vi "Manipulator Set Step.vi"(8 "error in (no error)":errorcluster, 10 "Step":i32, 11 "VISA resource in":refnum<visa-resource-name>="COM1") -> (0 "error out":errorcluster, 2 "Response":string, 3 "VISA resource out":refnum<visa-resource-name>)   [LabVIEW 2012, in "Scientifica Manipulator Daemon.lvlib"]
uses:
  Scientifica Manipulator Daemon.lvlib
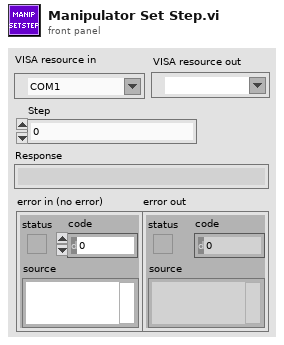
[diagram p1: front panel]
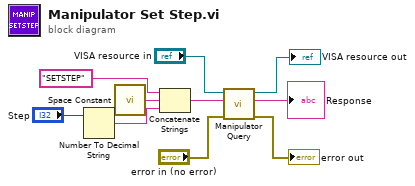
[diagram p0: block diagram]
diagram:
  n1 = Number To Decimal String(number="Step") -> (decimal integer string=w4:string)  [unwired: 1 in]
  n2 = call <vilib>:"Space Constant.vi"() -> ("String"=w5:string)
  n3 = Concatenate Strings("SETSTEP", w5, w4) -> (w3:string)
  n4 = call "Manipulator Query.vi"("error in (no error)"="error in (no error)", "Command"=w3, "VISA resource in"="VISA resource in") -> ("error out"=→"error out":errorcluster, "Response"=→"Response":string, "VISA resource out"=→"VISA resource out":refnum<visa-resource-name>)  [unwired: 5 in, 1 out]
